vi "9610 Missing mandatory sub-index--error.vi"(8 "error in (no error)":errorcluster, 10 "Sub-Index":u16, 11 "Index":u16) -> (0 "error out":errorcluster)   [LabVIEW 2024, in "Electronic Datasheet.lvlib"]
uses:
  Electronic Datasheet.lvlib
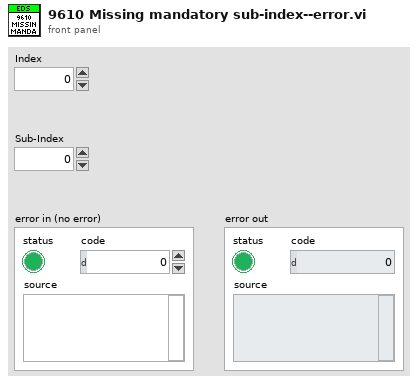
[diagram p1: front panel]
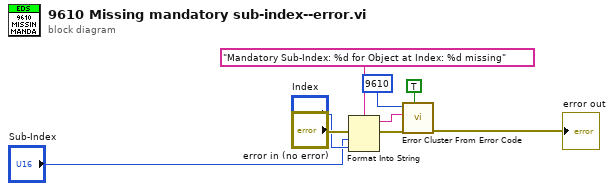
[diagram p0: block diagram]
diagram:
  n1 = Format Into String(format string="Mandatory Sub-Index: %d for Object at Index: %d missing", error in="error in (no error)", "Sub-Index", "Index") -> (resulting string=w3:string, error out=w4:errorcluster)  [unwired: 1 in]
  n2 = call <vilib>:"Error Cluster From Error Code.vi"("show call chain? (False)"=TRUE, "error in (no error)"=w4, "error message (\"\")"=w3, "error code (0)"=9610) -> ("error out"=→"error out":errorcluster)  [unwired: 5 in]
